vi "prueba_dac.vi"() -> ()   [LabVIEW 2025]
panel:
  in  "F":u32
  out "Salida":u8
  in  "stop":bool
  out "Voltaje":dbl
  in  "Pin":u8=25 min=25 max=26
  in  "VISA resource name":refnum<visa-resource-name>
  out "error out":errorcluster
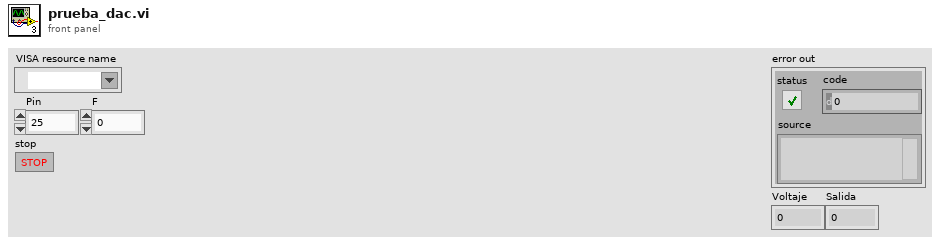
[diagram p1: front panel]
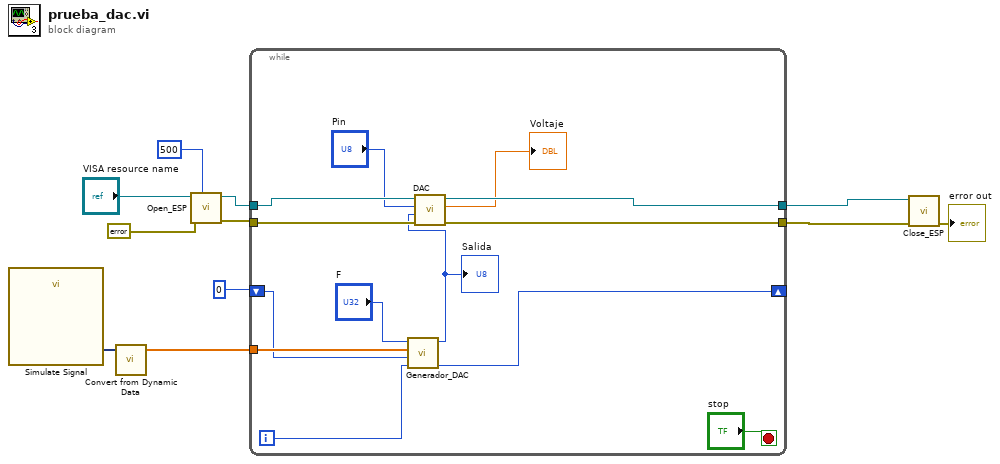
[diagram p0: block diagram]
diagram:
  n1 = call "Simulate Signal"() -> ("Sawtooth"=w3:dynamicdata)  [unwired: 14 in, 1 out]
  n2 = call "Convert from Dynamic Data"("Dynamic Data Type"=w3) -> ("Array"=w2:dbl[])  [unwired: 3 in]
  n3 = call "Open_ESP.vi"("timeout (10sec)"=u32 500, "error in (no error)"=errorcluster {"status"=FALSE, "code"=0, "source"=""}, "VISA resource name"="VISA resource name") -> ("error out"=w10:errorcluster, "VISA resource name out"=w11:refnum<visa-resource-name>)  [unwired: 7 in]
  n4 = while {
    tunnel: w11 -> [w24]
    tunnel: [w22] -> w9
    tunnel: w10 -> [w23]
    tunnel: [w21] -> w8
    tunnel: w2 -> [w17]
    shift-right: [w14] -> _
    shift-left: u32 0 ("timeout (10sec)") -> [w13]
    i -> [w16]
    stop <- "stop" stop-if-true
    n5 = call "Generador_DAC.vi"("Iteraciones"=w16, "entrada"=w13, "Entrada"=w17, "F"="F") -> ("salida_shift_reg"=w14:i64, "Salida"=w15:u8)  [unwired: 6 in]
    "Salida" <- w15
    n6 = call "DAC.vi"("error in (no error)"=w23, "DAC"=w15, "Pin"="Pin", "VISA resource name"=w24) -> ("error out"=w21:errorcluster, "Voltaje"=→"Voltaje":dbl, "VISA resource name out"=w22:refnum<visa-resource-name>)  [unwired: 5 in]
  }
  n7 = call "Close_ESP.vi"("error in (no error)"=w8, "VISA resource name"=w9) -> ("error out"=→"error out":errorcluster)  [unwired: 9 in]
